vi "PH_PPMA_PowerUnit.PC_StateDumpRods.vi"(0 "i ref in":refnum<vi>, 3 "Rods Status":T1 caption="Enabling State" items=["no info", "off/false/out", "on/true/in", "Failure", "Alarm", "Status 1", "Status 2", "Status 3"], 4 "not linked?":bool, 5 "error in (no error)":errorcluster) -> (14 "i ref out":refnum<vi> caption="VI Refnum", 19 "error out":errorcluster)   [LabVIEW 2014, in "PH_PPMA_PowerUnit.lvlib"]
doc: "This VI writes the Tag Information from the related Rods to own attributes, calculates the state of the device and sets the GUI object."
uses:
  PH_PPMA_PowerUnit.lvlib
  PH_StatusHandler/PH_StatusHandler.Status.ctl
  PH_Common/PH_Common.lvlib
  PH_PowerUnit_BaseClass/PH_PowerUnit_BaseClass.lvlib
  PH_StatusHandler/PH_StatusHandler.lvlib
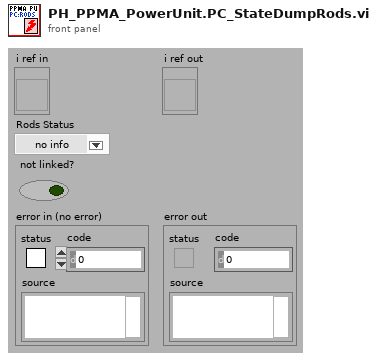
[diagram p1: front panel]
types:
  T1 = typedef "PH_StatusHandler.lvlib/PH_StatusHandler.Status.ctl" = i16
  T2 = typedef "PH_PowerUnit_BaseClass.lvlib/PH_PowerUnit_BaseClass.i attribute.ctl" = cluster{"Constructor finished":bool, "PU":cluster{"In use":bool, "Service ID in use":i32, "GUI Ref":refnum<vi>}, "Enabling":cluster{"State":T3, "GUI Ref":refnum<vi>}, "Timing":cluster{"Last Shot":dbl, "Time between Shots [Sec]":dbl, "Waiting Time over?":bool, "Service ID Waiting Time":i32, "GUI Ref":refnum<vi>, "Instance":cluster{"Status":T1, "linked?":bool, "GUI Ref":refnum<vi>}}, "Sequencer":cluster{"SM State":string, "GUI Ref":refnum<vi>, "linked":bool}, "Subscribed Trendmssgs":cluster{"Tagname":string, "Status":T1, "linked?":bool, "Shot Condition":T1, "GUI Ref":refnum<vi>}[], "PP PU":T4, "Default Voltage (V)":dbl, "GUI Refs":T5, "PSDB data":cluster{"Shot Voltage [V]":dbl, "State TO SM":T6, "Write 2 early":bool}, "State TO SM":T6}
  T3 = typedef "PH_SystemInformation.lvlib/PH_SystemInformationEnabling State.ctl" = i32
  T4 = typedef "PH_PP_Common.lvlib/PH_PP_Common.PUs.ctl" = enum16{"no Info", "PA-19mm-1", "PA-19mm-2", "PA-45mm-PILC", "PA-45mm-MAIN", "MA-PU-1", "MA-PU-2", "MA-PU-3", "MA-PU-4", "MA-PU-5", "MA-PU-6", "MA-FR", "MA-PILC", "PA-45mm-DP"}
  T5 = typedef "PH_PowerUnit_BaseClass.lvlib/PH_PowerUnit_BaseClass.GUI Refs.ctl" = cluster{"Delete Inst":refnum<vi>, "State TO SM":refnum<vi>, "State SM":refnum<vi>, "Fire":refnum<vi>}
  T6 = typedef "PH_PowerUnit_BaseClass.lvlib/PH_PowerUnit_BaseClass.SM States.ctl" = enum16{".", "Stand by", "Switch PU on", "Configure", "Set Default Voltage", "Set STANDBY", "Set READY", "Wait for Shot Cmd", "Open Dump Rods", "Open Ross Relais", "Close Ross Relais", "Switch PSU on", "Switch PSU off", "Charge", "Switch GD Channel on", "Close Dump Rods", "Rods-TO", "RR-TO", "PSU-TO", "Trigger-TO"}
  T7 = typedef "PH_PPMA_PowerUnit.lvlib/PH_PPMA_PowerUnit.i attribute.ctl" = cluster{"GUI Refs":cluster{"Rods":refnum<vi>, "Ignitron":refnum<vi>, "Rossrelais":refnum<vi>, "Set Voltage":refnum<vi>, "PSU":refnum<vi>, "EOC":refnum<vi>, "Trigger":refnum<vi>}, "Rods":T8, "PSU":T9, "Ross Relais":T10, "Ignitron":T11, "Trigger":cluster{"State Device":T1, "linked?":bool}, "Timing Settings":cluster{"Prdc Fast?":bool, "Default Value Periodic Interval":i32, "Mercury on since":dbl, "Warm up Time Mercury [s]":dbl}, "Set Voltage [V]":dbl}
  T8 = typedef "PH_PPMA_PowerUnit.lvlib/PH_PPMA_PowerUnit.Rods Attributes.ctl" = cluster{"Instancename":string, "Device Status":T1, "linked?":bool}
  T9 = typedef "PH_PP_Common.lvlib/PH_PP_Common.PSU Attributes.ctl" = cluster{"lower limit [V]":dbl, "upper limit [V]":dbl, "Voltage set":bool, "State Device":T1, "linked?":bool}
  T10 = typedef "PH_PP_Common.lvlib/PH_PP_Common.Ross Relais Attributes.ctl" = cluster{"State Device":T1, "linked?":bool}
  T11 = typedef "PH_PP_Common.lvlib/PH_PP_Common.Ignitron Attributes.ctl" = cluster{"State Device":T1, "linked?":bool}
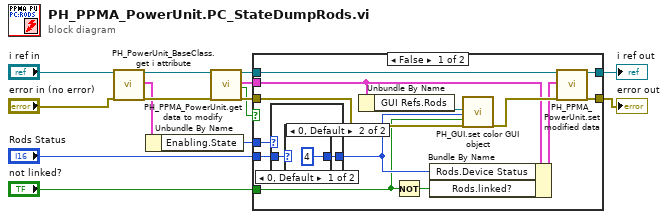
[diagram p0: block diagram]
diagram:
  n1 = call "PH_PowerUnit_BaseClass.get i attribute.vi"("i ref in"="i ref in", "error in (no error)"="error in (no error)") -> ("i ref out"=w3:refnum<vi>, "i attribute"=w2:T2, "error out"=w5:errorcluster)  [unwired: 15 in]
  n2 = Unbundle By Name(w2) -> ("Enabling.State"=w1:T3)
  n3 = call "PH_PPMA_PowerUnit.get data to modify.vi"("i ref in"=w3, "error in (no error)"=w5) -> ("i ref out"=w11:refnum<vi>, "i attribute"=w9:T7, "timed out"=w8:bool, "error out"=w10:errorcluster)  [unwired: 14 in]
  n4 = case shown="False" w8 {
    tunnel: w11 -> [w23 w34]
    tunnel: [w16 w34] -> w13
    tunnel: w10 -> [w27 w33]
    tunnel: [w17 w33] -> w14
    tunnel: w9 -> [w22 _]
    tunnel: "Rods Status" -> [w20 _]
    tunnel: "not linked?" -> [w19 _]
    tunnel: w1 -> [w15 _]
    frame False {
      n5 = case shown="0, Default" w15 {
        tunnel: w20 -> [w29 w32]
        tunnel: [w28 w32] -> w24
        frame 0, Default {
          n6 = case shown="0, Default" w29 {
            selector: w29 -> [w30 _]
            tunnel: [w30 i16 4] -> w28
            frame 1 {
            }
            frame 0, Default {
            }
          }
        }
        frame 1 {
        }
      }
      n7 = Unbundle By Name(w22) -> ("GUI Refs.Rods"=w21:refnum<vi>)
      n8 = Not(x=w19) -> (.not. x?=w18:bool)
      n9 = Bundle By Name(cluster=w22, "Rods.Device Status"=w24, "Rods.linked?"=w18) -> (w25:T7)
      n10 = call "PH_GUI.set color GUI object.vi"("GUI object Ref"=w21, "State"=w24, "Blinking? (false)"=w19, "error in (no error)"=w27) -> ("error out"=w26:errorcluster)  [unwired: 15 in]
      n11 = call "PH_PPMA_PowerUnit.set modified data.vi"("i ref in"=w23, "i attribute"=w25, "error in (no error)"=w26) -> ("i ref out"=w16:refnum<vi>, "error out"=w17:errorcluster)  [unwired: 15 in]
    }
    frame True {
    }
  }
  "error out" <- w14
  "i ref out" <- w13
